vi "New or edit user GUI.vi"(8 "error in (no error)":errorcluster, 9 "Edit index":i32, 10 "New user?":bool, 11 "Access Configuration in":T1 {"User array"."Expire sec" format="%.2f"}) -> (0 "error out":errorcluster, 1 "User ID":string, 2 "Cancelled?":bool, 3 "Access Configuration out":T1 {"User array"."Expire sec" format="%.2f"})   [LabVIEW 2013]
doc: "This is a pop-up panel which lets the system supervisor either add a new user (if \"New user?\" = T) or edit the existing user with \"Edit index\". It is a modal GUI.\n\nRequired input is the Access Configuration, which contains all the user access configuration parameters and current users.\n\nIf called with \"New user?\" = F the password fields are disabled. If \"New user?\" = T, then the \"Unlock and reset expiration?\" checkbox is not visable. The prompt also changes depending on the state of the \"new user?\" input.\n\nIf a new user, when the supervisor clicks Continue, the code:.\n1) checks that user ID field is not empty\n2) checks that the two new passwords are identical. If not, user is informed and the vi waits for another continue or cancel.\n3) If the two new passwords are equal, they are checked for minimum length of \"Min password char\" (from access configuration cluster) characters. If not of sufficient length, user is informed, and this vi waits for continue or cancel.\n4) the current time is used, along with the \"expire days\" setting from the access configuration cluster, to st the new user's expiration time.\n\nIf NOT a new user, when the supervisor clicks Continue, the code:.\n1) uses \"edit index\" to index the particular user's cluster from the input access configuration.\n2)checks if Active? checkbox is set, and sets corresponding field is user's config cluster.\n3) checks if the supervisor checked the reset checkbox, if set the user's locked and expired fields are cleared and new expiration time is set\n4) copies remaining fields to the user config."
uses:
  User Access Type defs/Security level U8.ctl
  User Access Type defs/Continue Button.ctl
  User Access Type defs/Cancel Button.ctl
  User Access Type defs/All users access configuration cluster.ctl
  User Access Type defs/User access cluster array.ctl
  User Access Type defs/User access cluster.ctl
panel:
  in  "Reset?":bool caption="Unlock account and/or reset expiration"
  in  "Security level":T4=5 max=10 step=1
  in  "New password 2":string caption="Password\n(repeat)"
  in  "Password":string
  in  "Full Name":string
  in  "User ID":string
  in  "Active?":bool
  out "State case":string
  in  "Cancel":T5
  in  "Continue":T6
  out "prompt":string="Edit the current user parameters and click Continue to save or Cancel to exit without saving"
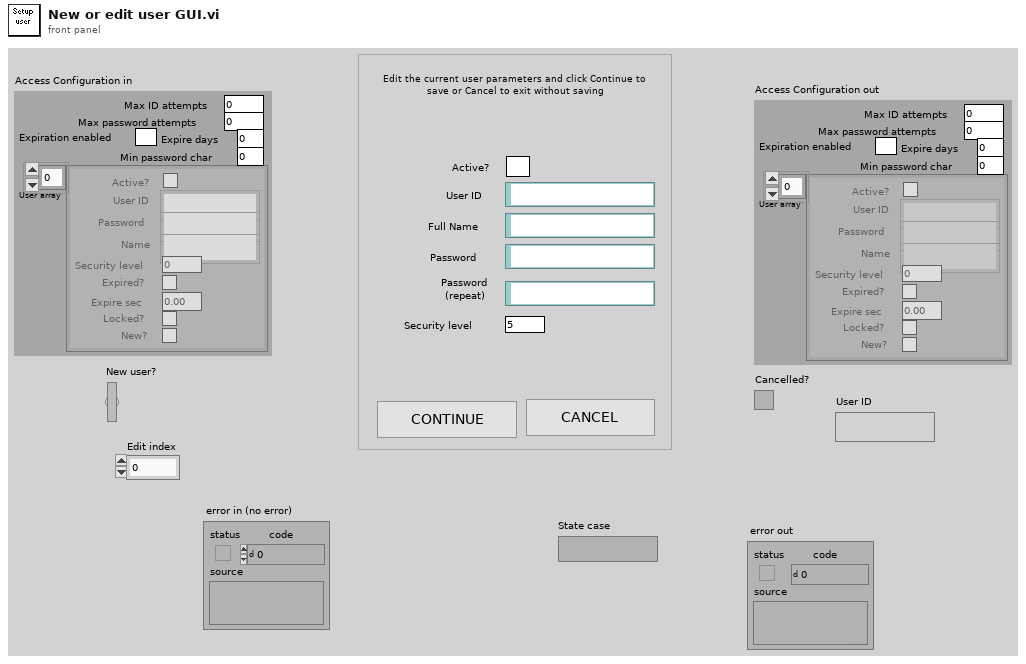
[diagram p1: front panel]
types:
  T1 = typedef "All users access configuration cluster.ctl" = cluster{"Max ID attempts":i32, "Max password attempts":i32, "Expiration enabled":bool, "Expire days":i32, "User array":T2, "Min password char":i32}
  T2 = typedef "User access cluster array.ctl" = T3[]
  T3 = typedef "User access cluster.ctl" = cluster{"Active?":bool, "User ID":string, "Password":string, "Name":string, "Security level":T4, "Expired?":bool, "Expire sec":dbl, "Locked?":bool, "New?":bool}
  T4 = typedef "Security level U8.ctl" = u8
  T5 = typedef "Cancel Button.ctl" = bool
  T6 = typedef "Continue Button.ctl" = bool
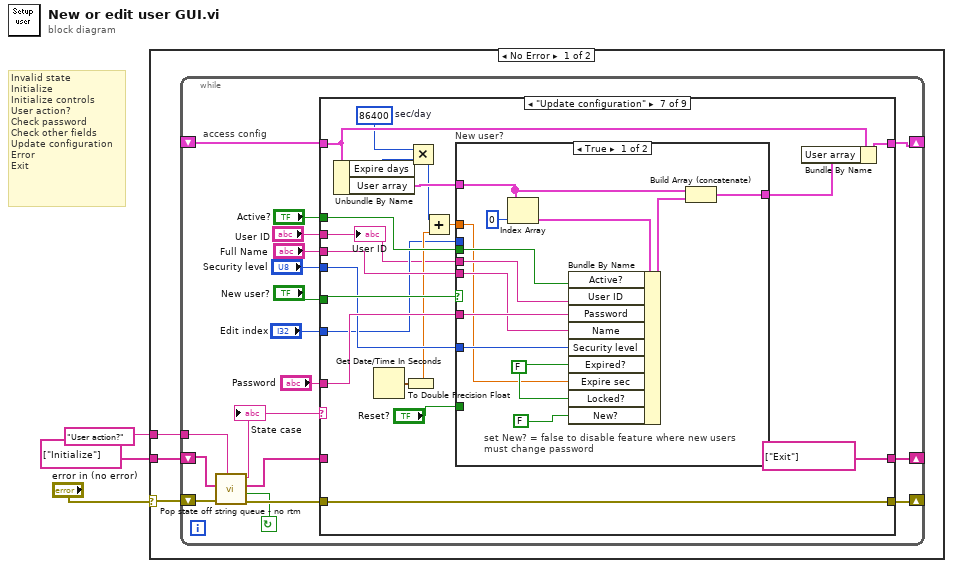
[diagram p0: block diagram]
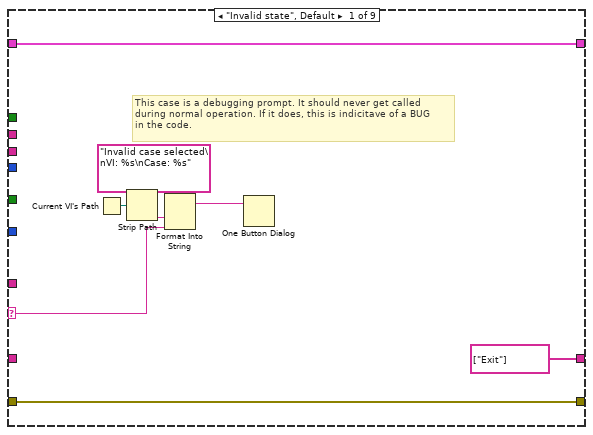
[diagram p2: hidden frame]
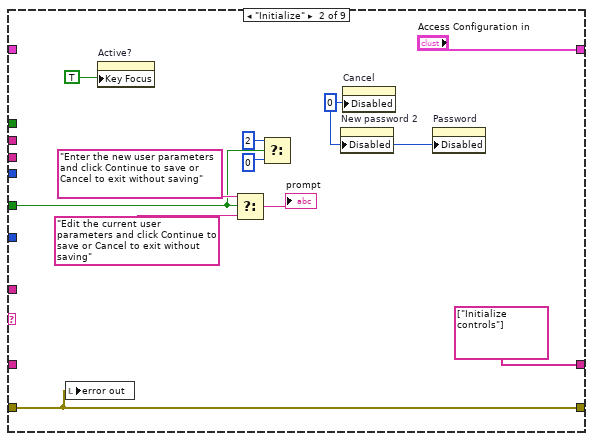
[diagram p3: hidden frame]
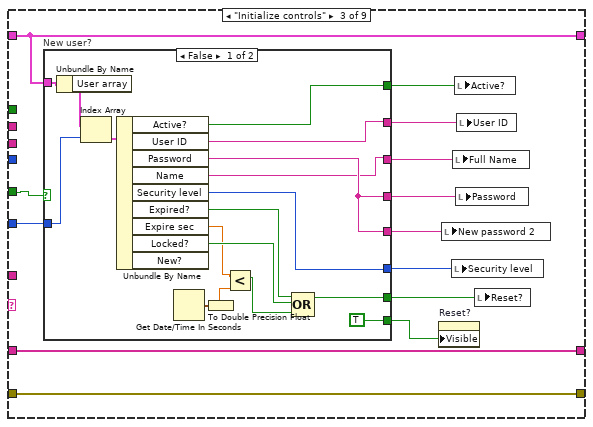
[diagram p4: hidden frame]
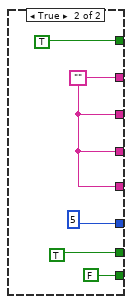
[diagram p5: hidden frame]
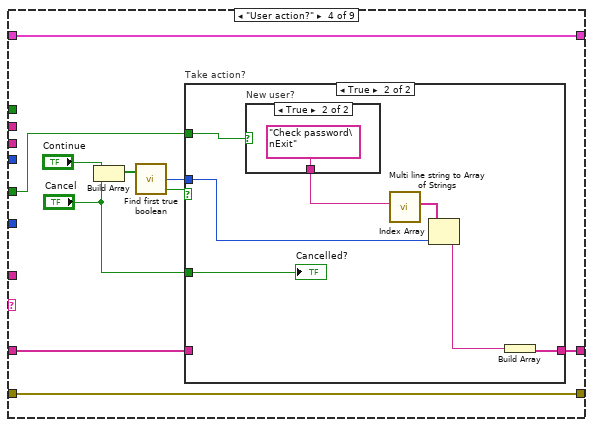
[diagram p6: hidden frame]
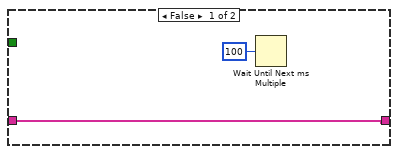
[diagram p7: hidden frame]
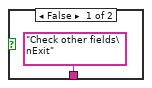
[diagram p8: hidden frame]
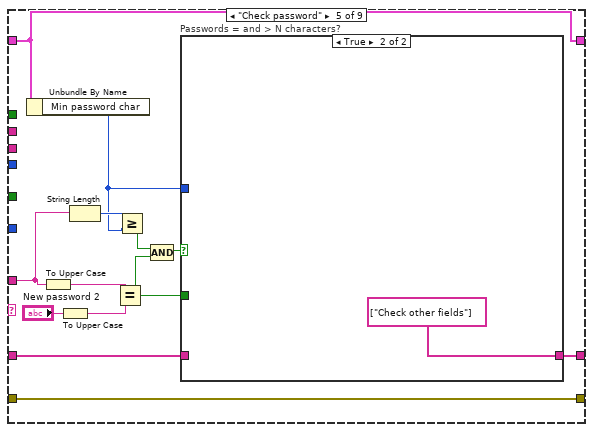
[diagram p9: hidden frame]
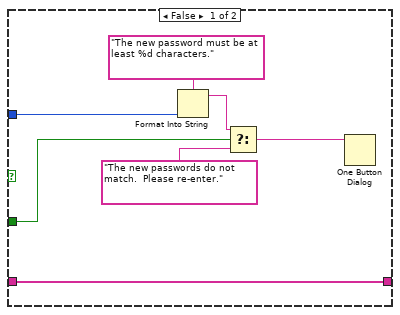
[diagram p10: hidden frame]
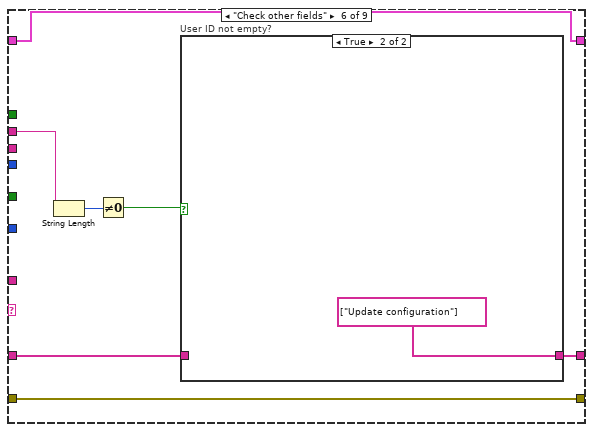
[diagram p11: hidden frame]
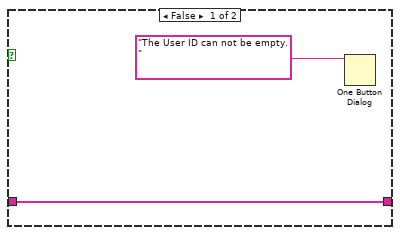
[diagram p12: hidden frame]
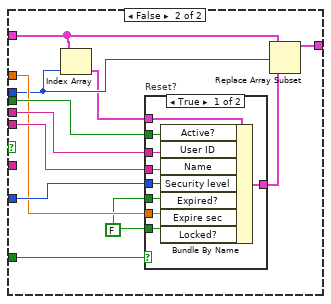
[diagram p13: hidden frame]
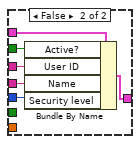
[diagram p14: hidden frame]
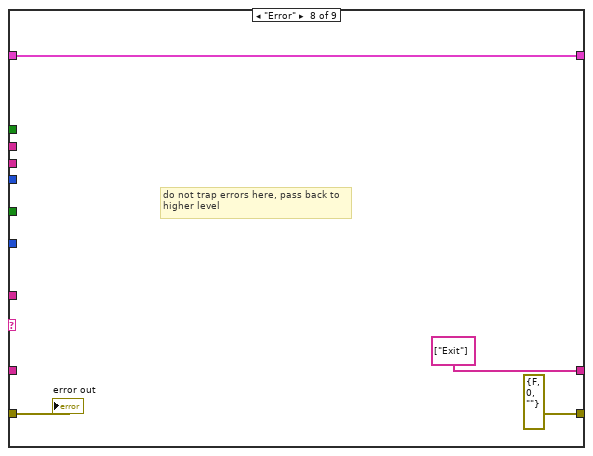
[diagram p15: hidden frame]
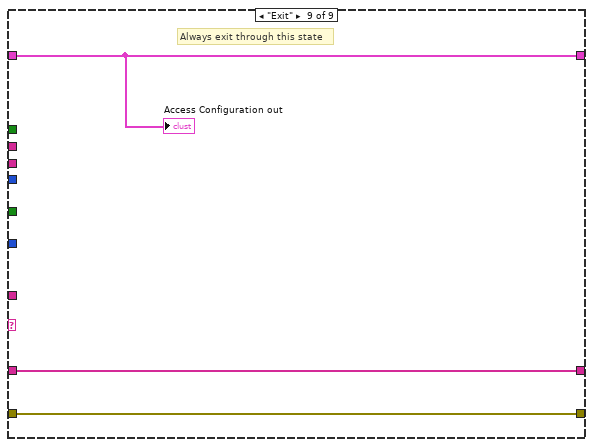
[diagram p16: hidden frame]
diagram:
  # "Invalid state\nInitialize\nInitialize controls\nUser action?\nCheck password\nCheck other fields\nUpdate configuration\nError\nExit"
  n1 = case shown="No Error" "error in (no error)" {
    selector: "error in (no error)" -> [w6 _]
    tunnel: string[] ["Initialize"] ("State que out") -> [w5 _]
    tunnel: "User action?" ("Default state") -> [w4 _]
    frame No Error {
      n2 = while {
        tunnel: w4 -> [w16]
        shift-left: w5 -> [w20]
        shift-right: [w18] -> _
        shift-left: w6 -> [w24]
        shift-right: [w22] -> _
        shift-right: [w14] -> _
        shift-left: _ -> [w15]
        stop <- w17 continue-if-true
        # "access config"
        n3 = call "Pop state off string queue - no rtm.vi"("Default state"=w16, "error in (no error)"=w24, "State que in"=w20) -> ("error out"=w23:errorcluster, "Not Exit?"=w17:bool, "State que out"=w19:string[], "State case"=w21:string)  [unwired: 5 out]
        "State case" <- w21
        n4 = case shown="\"Update configuration\"" w21 {
          selector: w21 -> [w27 _ _ _ _ _ _ _ _]
          tunnel: [w32 w43 w56 w88 w112 w127 w147 errorcluster {"status"=FALSE, "code"=0, "source"=""} ("error out") w196] -> w22
          tunnel: w23 -> [w32 w43 w56 w88 w112 w127 w147 w192 w196]
          tunnel: [string[] ["Exit"] ("State que out") string[] ["Initialize controls"] ("State que out") w55 w87 w111 w126 string[] ["Exit"] ("State que out") string[] ["Exit"] ("State que out") w197] -> w18
          tunnel: w19 -> [_ _ w55 w81 w109 w124 _ _ w197]
          tunnel: [w25 "Access Configuration in" w46 w86 w110 w125 w148 w191 w195] -> w14
          tunnel: w15 -> [w25 _ w46 w86 w110 w125 w149 w191 w195]
          tunnel: "New user?" -> [_ w36 w54 w80 _ _ w146 _ _]
          tunnel: "Password" -> [_ _ _ _ w106 _ w143 _ _]
          tunnel: "Edit index" -> [_ _ w45 _ _ _ w134 _ _]
          tunnel: "User ID" -> [_ _ _ _ _ w123 w132 _ _]
          tunnel: "Active?" -> [_ _ _ _ _ _ w144 _ _]
          tunnel: "Full Name" -> [_ _ _ _ _ _ w142 _ _]
          tunnel: "Security level" -> [_ _ _ _ _ _ w141 _ _]
          frame "Invalid state", Default {
            # "This case is a debugging prompt. It should never get called\nduring normal operation. If it does, this is indicitave of a BUG\nin the code."
            n5 = Current VI's Path() -> (path=w29:path)
            n6 = Strip Path(path=w29) -> (name=w28:string)  [unwired: 1 out]
            n7 = Format Into String(format string="Invalid case selected\nVI: %s\nCase: %s" ("message"), w28, w27) -> (resulting string=w30:string)  [unwired: 2 in, 1 out]
            n8 = One Button Dialog(message=w30) -> ()  [unwired: 2 out]
          }
          frame "Initialize" {
            w33 = u8 0 ("Disabled")
            n9 = local write "error out"(w43) -> ()
            n10 = property on="Active?" class="Bool (strict)"("Key Focus"=TRUE) -> ()  [unwired: 2 in, 2 out]
            n11 = Select(t="Enter the new user parameters and click Continue to save or Cancel to exit without saving" ("prompt"), s=w36, f="Edit the current user parameters and click Continue to save or Cancel to exit without saving" ("prompt")) -> (s? t:f=→"prompt":string)
            n12 = Select(t=u8 2 ("Disabled"), s=w36, f=u8 0 ("Disabled")) -> ()  [unwired: 1 out]
            n13 = property on="New password 2" class="Str"("Disabled"=w33) -> ()  [unwired: 2 in, 2 out]
            n14 = property on="Cancel" class="Bool"("Disabled"=w33) -> ()  [unwired: 2 in, 2 out]
            n15 = property on="Password" class="Str"("Disabled"=w33) -> ()  [unwired: 2 in, 2 out]
          }
          frame "Initialize controls" {
            n16 = case "New user?" shown="False" w54 {
              tunnel: [w61 w78] -> w53
              tunnel: [w62 w78] -> w52
              tunnel: [w63 w78] -> w51
              tunnel: [w63 w78] -> w50
              tunnel: [w60 TRUE] -> w49
              tunnel: [w59 TRUE] -> w48
              tunnel: [w64 T4 5 ("Security level")] -> w47
              tunnel: w46 -> [w73 _]
              tunnel: w45 -> [w71 _]
              tunnel: [TRUE FALSE] -> w44
              frame False {
                n17 = Unbundle By Name(w73) -> ("User array"=w72:T2)
                n18 = Index Array(array=w72, index=w71) -> (element=w70:T3)
                n19 = Unbundle By Name(w70) -> ("Active?"=w60:bool, "User ID"=w61:string, "Password"=w63:string, "Name"=w62:string, "Security level"=w64:T4, "Expired?"=w69:bool, "Expire sec"=w67:dbl, "Locked?"=w68:bool)  [unwired: 1 out]
                n20 = Get Date/Time In Seconds() -> (seconds since 1Jan1904=w57:timestamp)
                n21 = To Double Precision Float(number=w57) -> (double precision float=w66:dbl)
                n22 = Less?(x=w67, y=w66) -> (x < y?=w65:bool)
                n23 = Compound Arithmetic op=OR(w69, w68, w65) -> (w59:bool)
              }
              frame True {
                w78 = ""
              }
            }
            n24 = property on="Reset?" class="Bool (strict)"("Visible"=w44) -> ()  [unwired: 2 in, 2 out]
            n25 = local write "New password 2"(w51) -> ()
            n26 = local write "Security level"(w47) -> ()
            n27 = local write "Full Name"(w52) -> ()
            n28 = local write "Active?"(w49) -> ()
            n29 = local write "Password"(w50) -> ()
            n30 = local write "User ID"(w53) -> ()
            n31 = local write "Reset?"(w48) -> ()
          }
          frame "User action?" {
            n32 = Build Array("Continue", "Cancel") -> (w84:T5[])
            n33 = call "Find first true boolean.vi"("Boolean Array IN"=w84) -> ("Index of first (T)"=w82:i32, "True found?"=w83:bool)  [unwired: 2 out]
            n34 = case "Take action?" shown="True" w83 {
              tunnel: [w90 w94] -> w87
              tunnel: w82 -> [_ w96]
              tunnel: w81 -> [w90 _]
              tunnel: w80 -> [_ w92]
              tunnel: "Cancel" -> [_ w91]
              frame False {
                n35 = Wait Until Next ms Multiple(millisecond multiple=u32 100) -> ()  [unwired: 1 out]
              }
              frame True {
                n36 = case "New user?" shown="True" w92 {
                  tunnel: ["Check other fields\nExit" ("Multi Line String") "Check password\nExit" ("Multi Line String")] -> w93
                  frame False {
                  }
                  frame True {
                  }
                }
                n37 = call "Multi line string to Array of Strings.vi"("Multi Line String"=w93) -> ("Array of Strings"=w97:string[])  [unwired: 6 out]
                n38 = Index Array(array=w97, index=w96) -> (element=w95:string)
                n39 = Build Array(w95) -> (w94:string[])
                "Cancelled?" <- w91
              }
            }
          }
          frame "Check password" {
            n40 = Unbundle By Name(w110) -> ("Min password char"=w102:i32)
            n41 = To Upper Case(1:w106) -> (0:w100:string)
            n42 = To Upper Case(1:"New password 2") -> (0:w101:string)
            n43 = String Length(string=w106) -> (length=w105:i32)
            n44 = Equal?(x=w100, y=w101) -> (x = y?=w104:bool)
            n45 = Greater Or Equal?(x=w105, y=w102) -> (x >= y?=w108:bool)
            n46 = Compound Arithmetic op=AND(w108, w104) -> (w103:bool)
            n47 = case "Passwords = and > N characters?" shown="True" w103 {
              tunnel: [w119 string[] ["Check other fields"] ("State que out")] -> w111
              tunnel: w109 -> [w119 _]
              tunnel: w104 -> [w118 _]
              tunnel: w102 -> [w117 _]
              frame False {
                n48 = Format Into String(format string="The new password must be at least %d characters." ("message"), w117) -> (resulting string=w114:string)  [unwired: 2 in, 1 out]
                n49 = Select(t=w114, s=w118, f="The new passwords do not match.  Please re-enter." ("message")) -> (s? t:f=w116:string)
                n50 = One Button Dialog(message=w116) -> ()  [unwired: 2 out]
              }
              frame True {
              }
            }
          }
          frame "Check other fields" {
            n51 = String Length(string=w123) -> (length=w122:i32)
            n52 = Not Equal To 0?(x=w122) -> (x != 0?=w121:bool)
            n53 = case "User ID not empty?" shown="True" w121 {
              tunnel: [w129 string[] ["Update configuration"] ("State que out")] -> w126
              tunnel: w124 -> [w129 _]
              frame False {
                n54 = One Button Dialog(message="The User ID can not be empty.") -> ()  [unwired: 2 out]
              }
              frame True {
              }
            }
          }
          frame "Update configuration" {
            w139 = 86400  # sec/day
            n55 = Unbundle By Name(w149) -> ("Expire days"=w140:i32, "User array"=w145:T2)
            n56 = Get Date/Time In Seconds() -> (seconds since 1Jan1904=w131:timestamp)
            n57 = To Double Precision Float(number=w131) -> (double precision float=w137:dbl)
            n58 = Multiply(x=w139, y=w140) -> (x*y=w138:i32)
            n59 = Add(x=w138, y=w137) -> (x+y=w136:dbl)
            n60 = case "New user?" shown="True" w146 {
              tunnel: w145 -> [w153 w170]
              tunnel: w144 -> [w161 w175]
              tunnel: w132 -> [w160 w174]
              tunnel: w143 -> [w159 _]
              tunnel: w142 -> [w158 w173]
              tunnel: w141 -> [w157 w172]
              tunnel: w136 -> [w154 w171]
              tunnel: [w151 w169] -> w135
              tunnel: w134 -> [_ w167]
              tunnel: "Reset?" -> [_ w165]
              frame True {
                w156 = FALSE ("Expired?")
                # "set New? = false to disable feature where new users\nmust change password"
                n61 = Index Array(array=w153, index=0) -> (element=w162:T3)
                n62 = Bundle By Name(cluster=w162, "Active?"=w161, "User ID"=w160, "Password"=w159, "Name"=w158, "Security level"=w157, "Expired?"=w156, "Expire sec"=w154, "Locked?"=w156, "New?"=FALSE) -> (w152:T3)
                n63 = Build Array (concatenate)(w153, w152) -> (w151:T2)
              }
              frame False {
                w164 = FALSE ("Locked?")
                n64 = Index Array(array=w170, index=w167) -> (element=w166:T3)
                n65 = case "Reset?" shown="True" w165 {
                  tunnel: w175 -> [w184 w190]
                  tunnel: w174 -> [w183 w189]
                  tunnel: w173 -> [w182 w188]
                  tunnel: w172 -> [w181 w187]
                  tunnel: w171 -> [w180 _]
                  tunnel: [w179 w186] -> w168
                  tunnel: w166 -> [w178 w185]
                  tunnel: w164 -> [w177 _]
                  tunnel: w164 -> [w176 _]
                  frame True {
                    n66 = Bundle By Name(cluster=w178, "Active?"=w184, "User ID"=w183, "Name"=w182, "Security level"=w181, "Expired?"=w176, "Expire sec"=w180, "Locked?"=w177) -> (w179:T3)
                  }
                  frame False {
                    n67 = Bundle By Name(cluster=w185, "Active?"=w190, "User ID"=w189, "Name"=w188, "Security level"=w187) -> (w186:T3)
                  }
                }
                n68 = Replace Array Subset(array=w170, new element=w168, index=w167) -> (w169:T2)
              }
            }
            n69 = Bundle By Name(cluster=w149, "User array"=w135) -> (w148:T1)
            "User ID" <- w132
          }
          frame "Error" {
            # "do not trap errors here, pass back to\nhigher level"
            "error out" <- w192
          }
          frame "Exit" {
            # "Always exit through this state"
            "Access Configuration out" <- w195
          }
        }
      }
    }
    frame Error {
    }
  }
